vi "Not Equivalent Test.vi"() -> ()   [LabVIEW 2017]
uses:
  JSONtext.lvlib
  <vilib>/addons/_JKI Toolkits/Caraya/classes/Assert/Assert.lvclass
  <vilib>/addons/_JKI Toolkits/Caraya/classes/Test/Test.lvclass
panel:
  out "Not Equal":bool[](array[boolean])
  out "Equal":bool[](array[boolean])
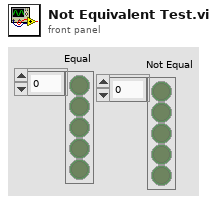
[diagram p1: front panel]
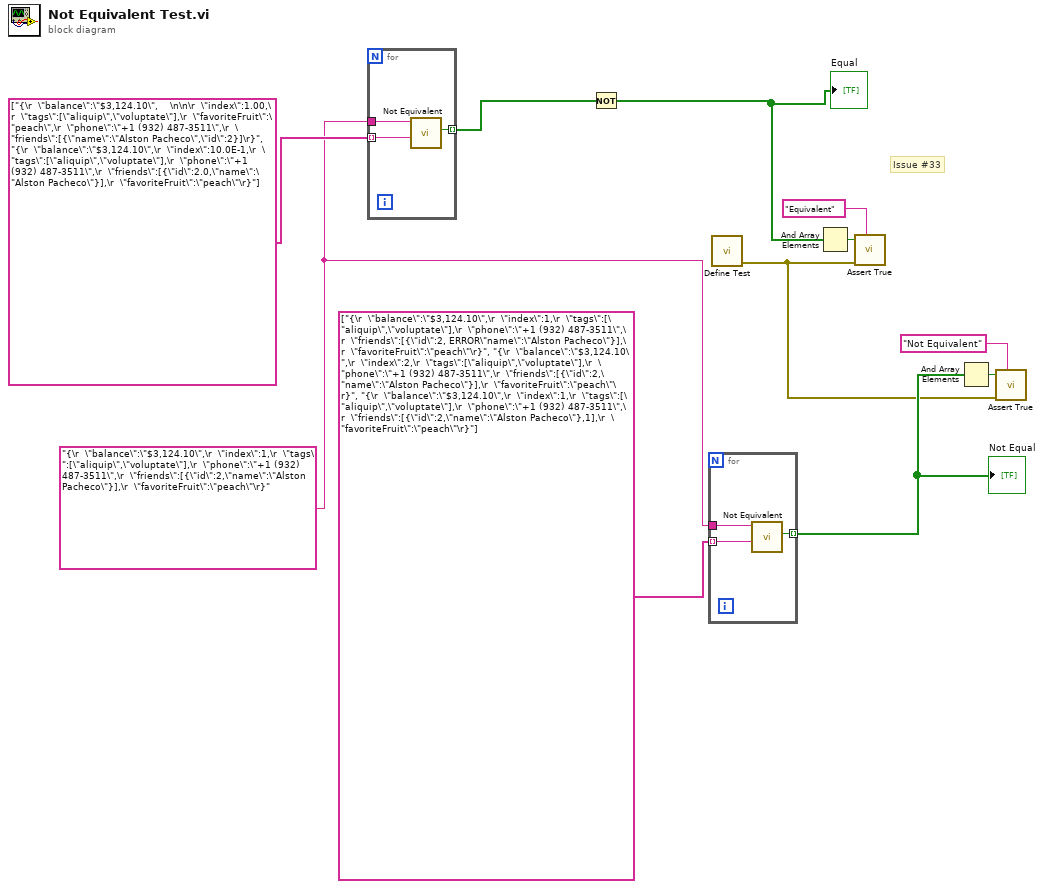
[diagram p0: block diagram]
diagram:
  w8 = "{\r  \"balance\":\"$3,124.10\",\r  \"index\":1,\r  \"tags\":[\"aliquip\",\"voluptate\"],\r  \"phone\":\"+1 (932) 487-3511\",\r  \"friends\":[{\"id\":2,\"name\":\"Alston Pacheco\"}],\r  \"favoriteFruit\":\"peach\"\r}" ("JSON Object")
  # "Issue #33"
  n1 = for {
    tunnel: w8 -> [w14]
    tunnel: [w13] -> w4 mode=indexing
    tunnel: string[] ["{\r  \"balance\":\"$3,124.10\",    \n\n\r  \"index\":1.00,\r  \"tags\":[\"aliquip\",\"voluptate\"],\r  \"favoriteFruit\":\"peach\",\r  \"phone\":\"+1 (932) 487-3511\",\r  \"friends\":[{\"name\":\"Alston Pacheco\",\"id\":2}]\r}", "{\r  \"balance\":\"$3,124.10\",\r  \"index\":10.0E-1,\r  \"tags\":[\"aliquip\",\"voluptate\"],\r  \"phone\":\"+1 (932) 487-3511\",\r  \"friends\":[{\"id\":2.0,\"name\":\"Alston Pacheco\"}],\r  \"favoriteFruit\":\"peach\"\r}"] ("JSON Object") -> [w12] mode=indexing
    n2 = call "Not Equivalent.vi"("Other JSON"=w12, "JSON"=w14) -> ("Not Equivalent"=w13:bool)  [unwired: 8 in]
  }
  n3 = Not(x=w4) -> (.not. x?=w3:bool[])
  "Equal" <- w3
  n4 = for {
    tunnel: w8 -> [w17]
    tunnel: [w16] -> w2 mode=indexing
    tunnel: string[] ["{\r  \"balance\":\"$3,124.10\",\r  \"index\":1,\r  \"tags\":[\"aliquip\",\"voluptate\"],\r  \"phone\":\"+1 (932) 487-3511\",\r  \"friends\":[{\"id\":2, ERROR\"name\":\"Alston Pacheco\"}],\r  \"favoriteFruit\":\"peach\"\r}", "{\r  \"balance\":\"$3,124.10\",\r  \"index\":2,\r  \"tags\":[\"aliquip\",\"voluptate\"],\r  \"phone\":\"+1 (932) 487-3511\",\r  \"friends\":[{\"id\":2,\"name\":\"Alston Pacheco\"}],\r  \"favoriteFruit\":\"peach\"\r}", "{\r  \"balance\":\"$3,124.10\",\r  \"index\":1,\r  \"tags\":[\"aliquip\",\"voluptate\"],\r  \"phone\":\"+1 (932) 487-3511\",\r  \"friends\":[{\"id\":2,\"name\":\"Alston Pacheco\"},1],\r  \"favoriteFruit\":\"peach\"\r}"] ("JSON Object") -> [w15] mode=indexing
    n5 = call "Not Equivalent.vi"("Other JSON"=w15, "JSON"=w17) -> ("Not Equivalent"=w16:bool)  [unwired: 8 in]
  }
  "Not Equal" <- w2
  n6 = call <vilib>:"Define Test.vi"() -> ("error out"=w1:errorcluster)  [unwired: 11 in]
  n7 = And Array Elements(Boolean array=w3) -> (logical AND=w10:bool)
  n8 = call <vilib>:"Assert True.vi"("Label"="Equivalent", "error in (no error)"=w1, "True?"=w10) -> ()  [unwired: 8 in, 1 out]
  n9 = And Array Elements(Boolean array=w2) -> (logical AND=w5:bool)
  n10 = call <vilib>:"Assert True.vi"("Label"="Not Equivalent", "error in (no error)"=w1, "True?"=w5) -> ()  [unwired: 8 in, 1 out]
